vi "P841_Ctrl_Index.vi"(5 "OldVal":variant, 11 "NewVal":variant) -> (4 "Control out":refnum<vi>, 8 "P841 Out":T1)   [LabVIEW 2014]
uses:
  Type Defs/P841.ctl
panel:
  in  "P841":T1
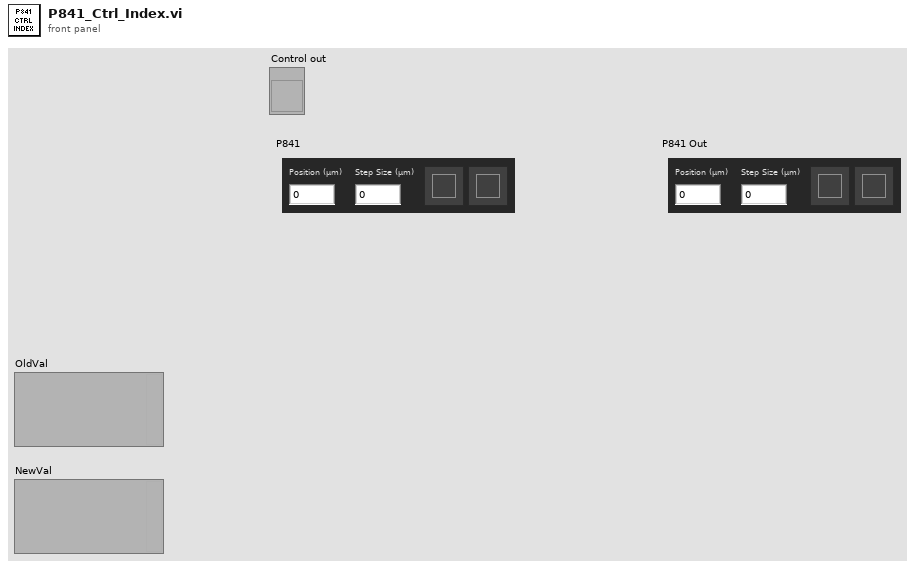
[diagram p1: front panel]
types:
  T1 = typedef "P841.ctl" = cluster{"Position (µm)":dbl, "Step Size (µm)":dbl, "Up P841":bool, "Down P841":bool}
  T2 = cluster{"Position (µm)":bool, "Step Size (µm)":bool, "Up P841":bool, "Down P841":bool}
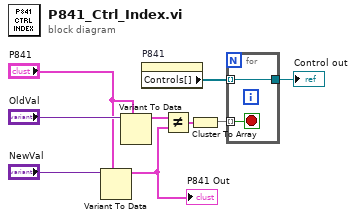
[diagram p0: block diagram]
diagram:
  n1 = Variant To Data(type="P841", Variant="NewVal") -> (data=w9:T1)  [unwired: 1 in, 1 out]
  "P841 Out" <- w9
  n2 = Variant To Data(type="P841", Variant="OldVal") -> (data=w4:T1)  [unwired: 1 in, 1 out]
  n3 = property on="P841" class="Clust"() -> ("Controls[]"=w1:refnum<vi>[])  [unwired: 2 in, 2 out]
  n4 = Not Equal?(x=w4, y=w9) -> (x != y?=w8:T2)
  n5 = Cluster To Array(cluster=w8) -> (array=w5:bool[])
  n6 = for {
    tunnel: w5 -> [w10] mode=indexing
    tunnel: w1 -> [w11] mode=indexing
    tunnel: [w11] -> w3
    stop <- w10 stop-if-true
  }
  "Control out" <- w3
